vi "MT Detect PSK.vi"(5 "input complex waveform":T3={"t0"=0.0, "dt"=1.0, "Y"=[]} {"Y" format="%.3f"; "dt" format="%^.2e"; "t0" format="%.4f"}, 7 "PSK system parameters":T2={"samples per symbol (16)"=16, "symbol map"=[], "differential PSK"=enum."disable", "PSK type"=0} {"PSK type" items=["normal", "shifted", "offset"]; "symbol map" format="%.3f"}, 9 "synchronization parameters":T1 {"sync sequence" format="%.2f"}, 11 "error in (no error)":errorcluster, 12 "matched filter coefficients":dbl[](array[numeric]) format="%.2f", 13 "reset? (T)":bool=TRUE, 14 "flush buffers? (F)":bool) -> (6 "output bit stream":i8[](array[numeric]), 10 "sync found index (symbols)":dbl format="%.4f", 15 "error out":errorcluster)   [LabVIEW 2020, in "niDMT.lvlib"]
doc: "Demodulates a phase-shift keying (PSK)-modulated complex baseband waveform and returns the demodulated bit stream. This VI attempts to remove carrier and phase offset by locking to the carrier signal."
uses:
  <vilib>/addons/Modulation/niDMT.lvlib
  <vilib>/addons/Modulation/Analog/controls/Complex Data Waveform.ctl
  <vilib>/Utility/error.llb/Error Cluster From Error Code.vi
  <vilib>/addons/Modulation/Digital/Support/Common/mod_Truncate FIR Filter (complex).vi
  <vilib>/addons/Modulation/niAMT.lvlib
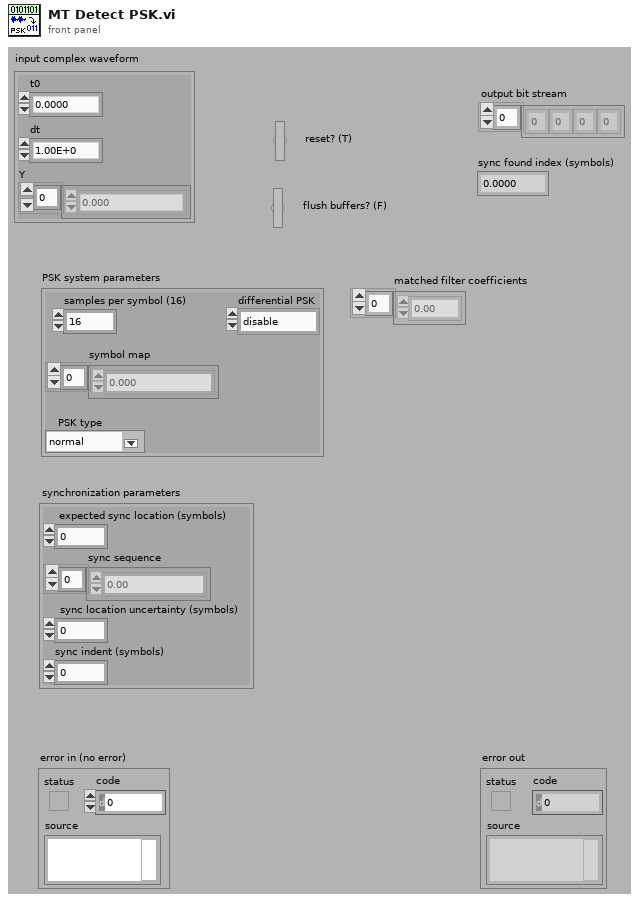
[diagram p1: front panel]
types:
  T1 = cluster{"expected sync location (symbols)":i32, "sync sequence":cdb[], "sync location uncertainty (symbols)":i32, "sync indent (symbols)":i32}
  T2 = cluster{"samples per symbol (16)":i32, "symbol map":cdb[], "differential PSK":enum16{"disable", "enable"}, "PSK type":u16}
  T3 = typedef "niAMT.lvlib/Complex Data Waveform.ctl" = cluster{"t0":dbl, "dt":dbl, "Y":cdb[]}
  T4 = cluster{"samples per symbol (16)":i32, "symbol map":cdb[], "differential PSK":enum16{"disable", "enable"}}
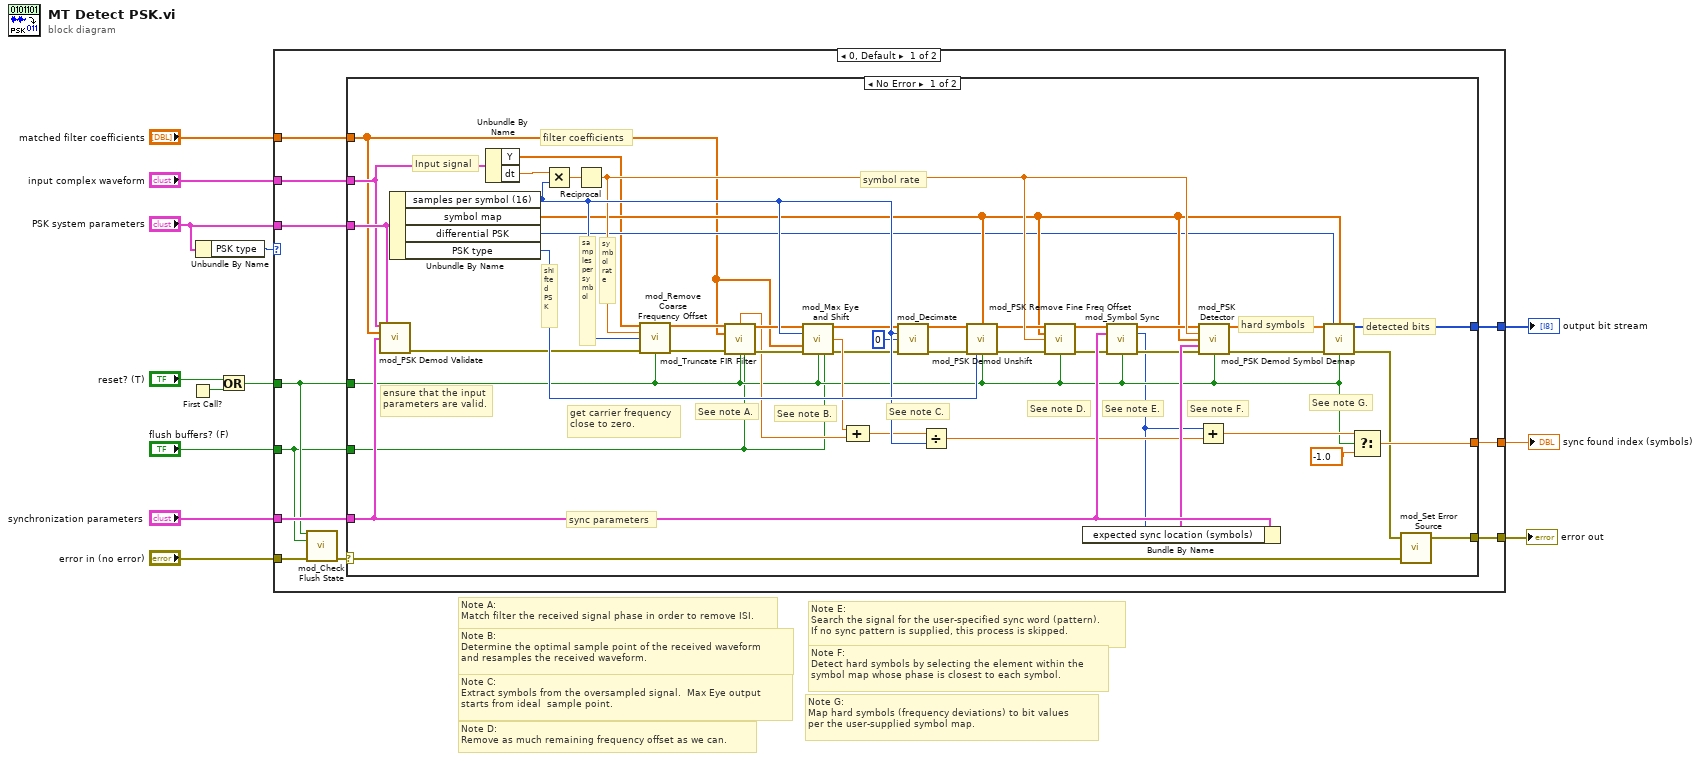
[diagram p0: block diagram]
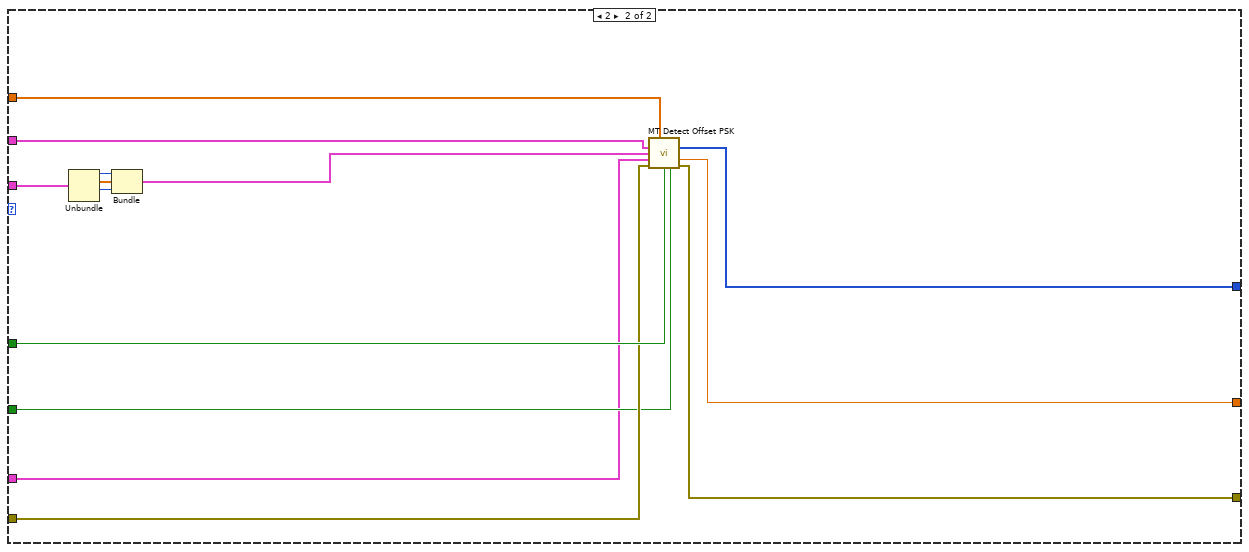
[diagram p3: hidden frame]
diagram:
  # "Note F:\nDetect hard symbols by selecting the element within the\nsymbol map whose phase is closest to each symbol."
  # "Note A:\nMatch filter the received signal phase in order to remove ISI."
  # "Note B:\nDetermine the optimal sample point of the received waveform \nand resamples the received waveform."
  # "Note C:\nExtract symbols from the oversampled signal.  Max Eye output \nstarts from ideal  sample point."
  # "Note D:\nRemove as much remaining frequency offset as we can."
  # "Note E:\nSearch the signal for the user-specified sync word (pattern).\nIf no sync pattern is supplied, this process is skipped."
  # "Note G:\nMap hard symbols (frequency deviations) to bit values \nper the user-supplied symbol map."
  n1 = First Call?() -> (First Call?: T/F=w6:bool)
  n2 = Unbundle By Name("PSK system parameters") -> ("PSK type"=w2:u16)
  n3 = Or(x="reset? (T)", y=w6) -> (x .or. y?=w4:bool)
  n4 = case shown="0, Default" w2 {
    tunnel: "error in (no error)" -> [w16 w79]
    tunnel: "input complex waveform" -> [w24 w72]
    tunnel: [w23 w78] -> w11
    tunnel: "matched filter coefficients" -> [w22 w71]
    tunnel: [w21 w74] -> w9
    tunnel: "synchronization parameters" -> [w20 w76]
    tunnel: [w19 w75] -> w7
    tunnel: w4 -> [w15 w80]
    tunnel: "PSK system parameters" -> [w18 w84]
    tunnel: "flush buffers? (F)" -> [w14 w77]
    frame 0, Default {
      # "normal and shifted case"
      n5 = call <vilib>:"mod_Check Flush State.vi"("reset?"=w15, "flush buffers? (F)"=w14, "error in (no error)"=w16) -> ("error out"=w17:errorcluster)  [unwired: 12 out]
      n6 = case shown="No Error" w17 {
        selector: w17 -> [w59 w70]
        tunnel: w15 -> [w35 _]
        tunnel: w24 -> [w63 _]
        tunnel: [w60 w70] -> w23
        tunnel: w22 -> [w30 _]
        tunnel: [w69 _] -> w19
        tunnel: [w67 _] -> w21
        tunnel: w18 -> [w64 _]
        tunnel: w20 -> [w62 _]
        tunnel: w14 -> [w26 _]
        frame No Error {
          # "filter coefficients"
          # "Input signal"
          # "ensure that the input parameters are valid."
          # "symbol rate"
          # "detected bits"
          # "hard symbols"
          # "sync parameters"
          # "samples per symbol"
          # "shifted PSK"
          # "See note A."
          # "See note B."
          # "ensure that the input parameters are valid."
          # "get carrier frequency close to zero."
          # "See note C."
          # "See note D."
          # "See note E."
          # "See note F."
          # "See note G."
          # "symbol rate"
          n7 = call <vilib>:"mod_PSK Demod Validate.vi"("Input Complex Waveform"=w63, "PSK System Parameters"=w64, "Matched Filter Coefficients"=w30, "Synchronization Parameters"=w62) -> ("error out"=w65:errorcluster)  [unwired: 3 in, 8 out]
          n8 = Unbundle By Name(w64) -> ("samples per symbol (16)"=w66:i32, "symbol map"=w32:cdb[], "differential PSK"=w31:enum16{"disable", "enable"}, "PSK type"=w68:u16)
          n9 = Unbundle By Name(w63) -> ("Y"=w29:cdb[], "dt"=w28:dbl)
          n10 = Multiply(x=w28, y=w66) -> (x*y=w55:dbl)
          n11 = Reciprocal(x=w55) -> (1/x=w49:dbl)
          n12 = call <vilib>:"mod_Remove Coarse Frequency Offset.vi"("Signal In"=w29, "Symbol Rate, Hz"=w49, "Samples Per Symbol (16)"=w66, "error in (no error)"=w65, "Reset? (T)"=w35) -> ("Signal Out"=w41:cdb[], "error out"=w58:errorcluster)  [unwired: 3 in, 6 out]
          n13 = call-poly <vilib>:"mod_Truncate FIR Filter.vi"("Signal In"=w41, "Filter Coefficients"=w30, "error in (no error)"=w58, "Reset? (T)"=w35, "flush buffers? (F)"=w26) -> ("Fractional Delay (samples)"=w39:dbl, "Signal Out"=w53:cdb[], "error out"=w52:errorcluster)  [unwired: 8 out]
          n14 = call <vilib>:"mod_Max Eye and Shift.vi"("Signal In"=w53, "Samples Per Symbol (16)"=w66, "matched filter coefficients"=w30, "error in (no error)"=w52, "Reset? (T)"=w35, "flush buffers? (F)"=w26) -> ("Signal Out"=w37:cdb[], "Optimal Offset (in Samples)"=w38:dbl, "error out"=w36:errorcluster)  [unwired: 7 out]
          n15 = Compound Arithmetic op=ADD(w38, w39) -> (w40:dbl)
          n16 = call <vilib>:"mod_Decimate.vi"("Signal In"=w37, "Samples Per Symbol (16)"=w66, "Offset"=0, "error in (no error)"=w36) -> ("Signal Out"=w44:cdb[], "error out"=w56:errorcluster)  [unwired: 10 out]
          n17 = Divide(x=w40, y=w66) -> (x/y=w54:dbl)
          n18 = call <vilib>:"mod_PSK Demod Unshift.vi"("Signal In"=w44, "Symbol Map"=w32, "error in (no error)"=w56, "Shifted PSK Enable (disable)"=w68, "Reset? (T)"=w35) -> ("Unshifted Signal"=w43:cdb[], "error out"=w48:errorcluster)  [unwired: 2 in, 7 out]
          n19 = call <vilib>:"mod_PSK Remove Fine Freq Offset.vi"("Symbols"=w43, "Symbol Map"=w32, "Symbol Rate, Hz"=w49, "error in (no error)"=w48, "Reset? (T)"=w35) -> ("Symbols"=w42:cdb[], "error out"=w47:errorcluster)  [unwired: 9 out]
          n20 = call <vilib>:"mod_Symbol Sync.vi"("Signal In"=w42, "Synchronization Parameters"=w62, "error in (no error)"=w47, "Reset? (T)"=w35) -> ("Signal Out"=w45:cdb[], "Sync Location (symbols)"=w27:i32, "error out"=w46:errorcluster)  [unwired: 1 in, 8 out]
          n21 = Bundle By Name(cluster=w62, "expected sync location (symbols)"=w27) -> (w57:T1)
          n22 = Add(x=w27, y=w54) -> (x+y=w51:dbl)
          n23 = call <vilib>:"mod_PSK Detector.vi"("Signal In"=w45, "Symbol Rate, Hz"=w49, "Symbol Map"=w32, "Synchronization Parameters"=w57, "error in (no error)"=w46, "Reset (T)"=w35) -> ("Signal Out"=w34:cdb[], "error out"=w33:errorcluster)  [unwired: 1 in, 7 out]
          n24 = call <vilib>:"mod_PSK Demod Symbol Demap.vi"("Symbols In"=w34, "Differential PSK Enable"=w31, "Symbol Map"=w32, "error in (no error)"=w33, "Reset? (T)"=w35) -> ("Bits Out"=w69:i8[], "error out"=w61:errorcluster)  [unwired: 1 in, 8 out]
          n25 = Select(t=w51, s=w35, f=-1.0) -> (s? t:f=w67:dbl)
          n26 = call <vilib>:"mod_Set Error Source.vi"("initial error in (no error)"=w59, "final error in (no error)"=w61) -> ("error out"=w60:errorcluster)  [unwired: 3 out]
        }
        frame Error {
        }
      }
    }
    frame 2 {
      # "offset case"
      n27 = Unbundle(w84) -> ("samples per symbol (16)"=w83:i32, "symbol map"=w82:cdb[], "differential PSK"=w81:enum16{"disable", "enable"})  [unwired: 1 out]
      n28 = Bundle("samples per symbol (16)"=w83, "symbol map"=w82, "differential PSK"=w81) -> (w73:T4)  [unwired: 1 out]
      n29 = call <vilib>:"MT Detect Offset PSK.vi"("input complex waveform"=w72, "Offset PSK system parameters"=w73, "synchronization parameters"=w76, "error in (no error)"=w79, "matched filter coefficients"=w71, "reset? (T)"=w80, "flush buffers? (F)"=w77) -> ("output bit stream"=w75:i8[], "sync found index (symbols)"=w74:dbl, "error out"=w78:errorcluster)  [unwired: 2 in, 4 out]
    }
  }
  "error out" <- w11
  "sync found index (symbols)" <- w9
  "output bit stream" <- w7
